vi "LV diagram subvis.vi"(8 "error in (no error)":errorcluster, 11 "reference":refnum<vi>) -> (3 "sUBvIS":string)   [LabVIEW 2012]
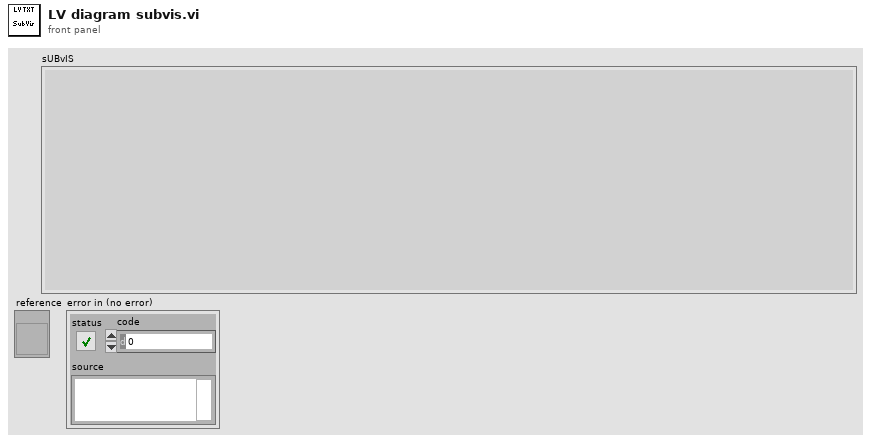
[diagram p1: front panel]
types:
  T1 = cluster{"UID":i32, "ClassID":u32, "ClassName":string, "Caption":string, "Name":string}
  T2 = cluster{"UID":i32, "ClassID":u32, "ClassName":string, "VIName":string, "VIPath":path, cluster{"UID":i32, "ClassID":u32, "ClassName":string, "Caption":string, "Name":string}[]}
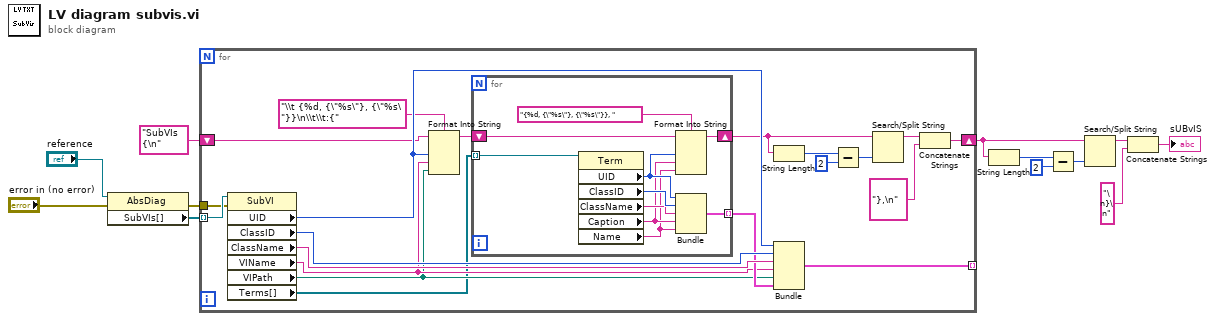
[diagram p0: block diagram]
diagram:
  n1 = property class="AbsDiag"(reference="reference", error in="error in (no error)") -> (error out=w11:errorcluster, "SubVIs[]"=w12:refnum<vi>[])  [unwired: 1 out]
  n2 = for {
    tunnel: w12 -> [w32] mode=indexing
    tunnel: [w29] -> _ mode=indexing
    tunnel: w11 -> [w27]
    shift-right: [w21] -> w4
    shift-left: "SubVIs {\n" ("format string") -> [w25]
    n3 = property class="SubVI"(reference=w32, error in=w27) -> ("UID"=w26:i32, "ClassID"=w31:u32, "ClassName"=w30:string, "VIName"=w15:string, "VIPath"=w14:path, "Terms[]"=w13:refnum<vi>[])  [unwired: 2 out]
    n4 = Format Into String(format string="\\t {%d, {\"%s\"}, {\"%s\"}}\n\\t\\t:{", initial string=w25, w26, w15, w14) -> (resulting string=w23:string)  [unwired: 1 in, 1 out]
    n5 = for {
      tunnel: w13 -> [w42] mode=indexing
      tunnel: [w41] -> w28 mode=indexing
      shift-right: [w37] -> w20
      shift-left: w23 -> [w38]
      n6 = property class="Term"(reference=w42) -> ("UID"=w40:i32, "ClassID"=w36:u32, "ClassName"=w35:string, "Caption"=w34:string, "Name"=w33:string)  [unwired: 1 in, 2 out]
      n7 = Format Into String(format string="{%d, {\"%s\"}, {\"%s\"}}, ", initial string=w38, w40, w34, w33) -> (resulting string=w37:string)  [unwired: 1 in, 1 out]
      n8 = Bundle("UID"=w40, "ClassID"=w36, "ClassName"=w35, "Caption"=w34, "Name"=w33) -> (w41:T1)  [unwired: 1 in]
    }
    n9 = String Length(string=w20) -> (length=w19:i32)
    n10 = Bundle("UID"=w26, "ClassID"=w31, "ClassName"=w30, "VIName"=w15, "VIPath"=w14, w28) -> (w29:T2)  [unwired: 1 in]
    n11 = Subtract(x=w19, y=2) -> (x-y=w17:i32)
    n12 = Search/Split String(string=w20, offset (0)=w17) -> (substring before match=w16:string)  [unwired: 1 in, 2 out]
    n13 = Concatenate Strings(w16, "},\n" ("format string")) -> (w21:string)
  }
  n14 = String Length(string=w4) -> (length=w5:i32)
  n15 = Subtract(x=w5, y=2) -> (x-y=w7:i32)
  n16 = Search/Split String(string=w4, offset (0)=w7) -> (substring before match=w3:string)  [unwired: 1 in, 2 out]
  n17 = Concatenate Strings(w3, "\n}\n" ("format string")) -> (→"sUBvIS":string)
